vi "xc_probe.vi"() -> ()   [LabVIEW 2014]
uses:
  PIXIS_TEST/SITK_Labview/Examples70_2_2_0_1/RS Pixis/MaxY.vi
  PIXIS_TEST/SITK_Labview/Examples70_2_2_0_1/RS Pixis/MaxX.vi
  <vilib>/Analysis/Matrix/Numeric/Conversions/Array To Matrix - RA.vi
  <vilib>/Analysis/Matrix/Numeric/Conversions/Array To Matrix - RA2.vi
  <vilib>/Math Plots/3D Math Plots/3D Surface/3D Surface Datatype/Public/Plot Helper (Matrix).vi
  <vilib>/Utility/file.llb/Write To Spreadsheet File (DBL).vi
  <vilib>/Utility/file.llb/Read From Spreadsheet File (DBL).vi
  <vilib>/Analysis/Matrix/NI_Matrix.lvlib
  <vilib>/Math Plots/3D Math Plots/3D Surface/3D Surface Datatype/3D Surface Datatype.lvclass
panel:
  out "Intensity Graph":dbl[][](graph)
  in  "Background":bool=TRUE
  in  "Filter":bool=TRUE
  in  "initial parameters":dbl[](array[numeric])
  in  "?":enum16{"Lorantzian", "fano", "gaussian"}(ring)=enum."gaussian"
  in  "parameter bounds":T1={"amp min"=-inf, "amp max"=inf, "deviation min"=-inf, "deviation max"=inf, "offset min"=0.0, "offset max"=0.0}
  in  "file path":path
  in  "fit":bool
  in  "pick":bool
  in  "quit Button 2":bool
  in  "# Images":u16=200 min=2 max=10000 step=2
  in  "Flip Spectra":bool
  out "Temperature":dbl=-75.5
  out "error out":errorcluster
  out "Camera Handle":u32=16842752
  in  "error in":errorcluster
  out "Waveform Graph":dbl[](graph)
  out "Identification":string="(c)2010 Physik Instrumente(PI) Karlsruhe, C-867.160,0,1.2.0.1"
  out "PI Stage Error 2":errorcluster
  in  "PI Stage Error":errorcluster
  in  "Shutter Position":bool=TRUE
  out "Status":string="Shutter Closed"
  in  "error in2":errorcluster
  out "error out 2":errorcluster={"status"=TRUE, "code"=1097, "source"="Call Library Function Node in Shutter_Close.vi->xc_umn1.vi"}
  out "Current position":dbl=9.0349
  in  "move":bool
  in  "Start Position":dbl=9.0
  in  "Averages":u16=2
  in  "save":bool
  in  "quit Button":bool
  in  "Start Button":bool
  in  "Increment (in mm)":dbl=0.01
  in  "Range (in mm)":dbl=6.0
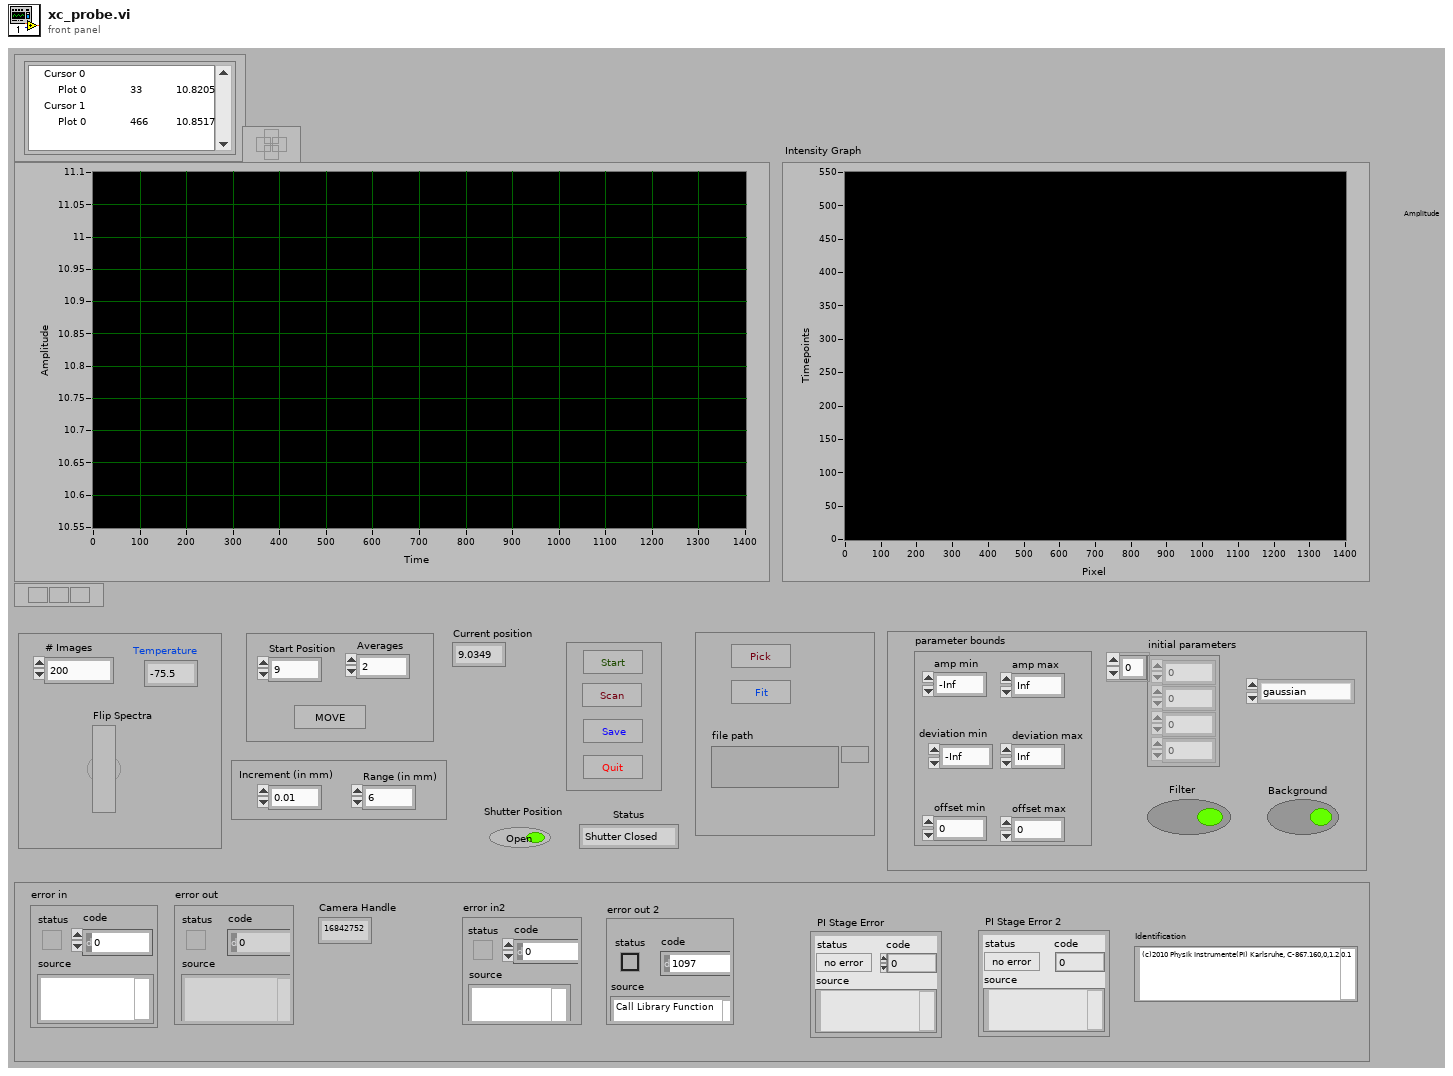
[diagram p1: front panel]
types:
  T1 = cluster{"amp min":dbl, "amp max":dbl, "deviation min":dbl, "deviation max":dbl, "offset min":dbl, "offset max":dbl}
  T2 = cluster{"X start":u32, "X end":u32, "X Binning/Grouping":u32, "Y start":u32, "Y end":u32, "Y Binning/Grouping":u32}
  T3 = typedef "NI_Matrix.lvlib/RealMatrix.ctl" = dbl[][]
  T4 = cluster{"amp min":dbl, "amp max":dbl, dbl, dbl, "deviation min":dbl, "deviation max":dbl, "offset min":dbl, "offset max":dbl}
  T5 = cluster{dbl, "result":dbl, dbl, "delta amplitude":dbl, dbl, "delta standard deviation":dbl, "center":dbl, "delta center":dbl}
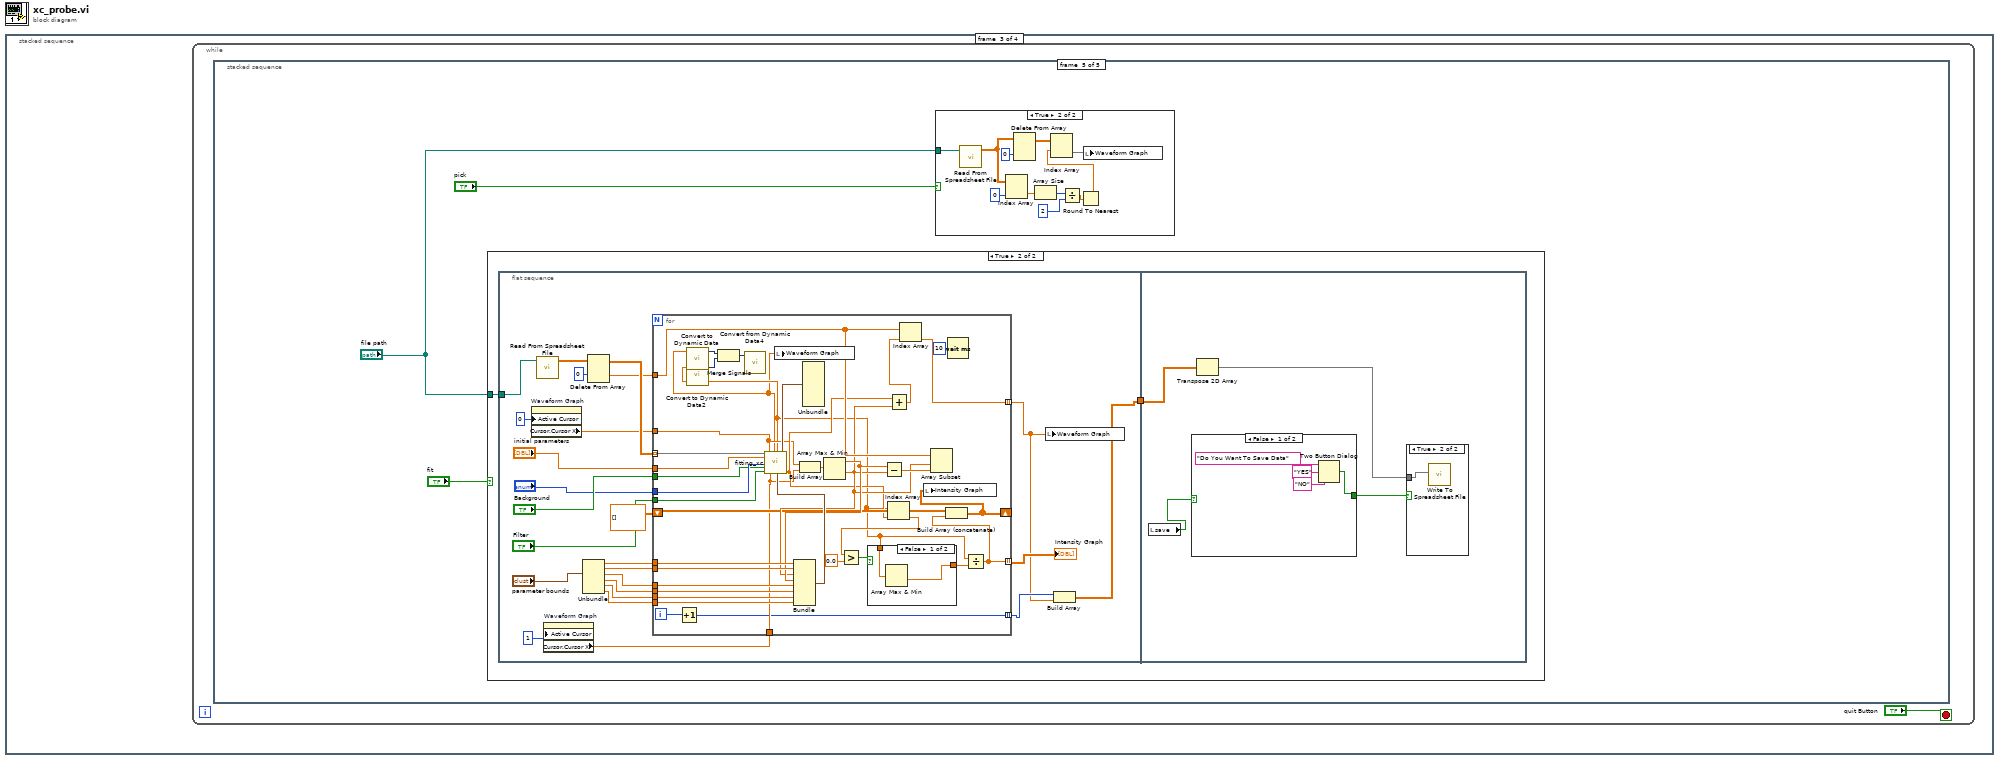
[diagram p0: block diagram]
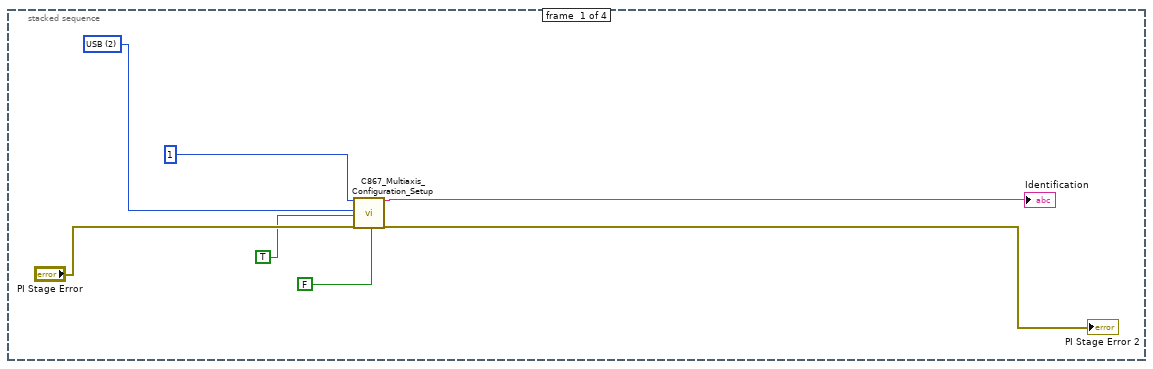
[diagram p2: hidden frame]
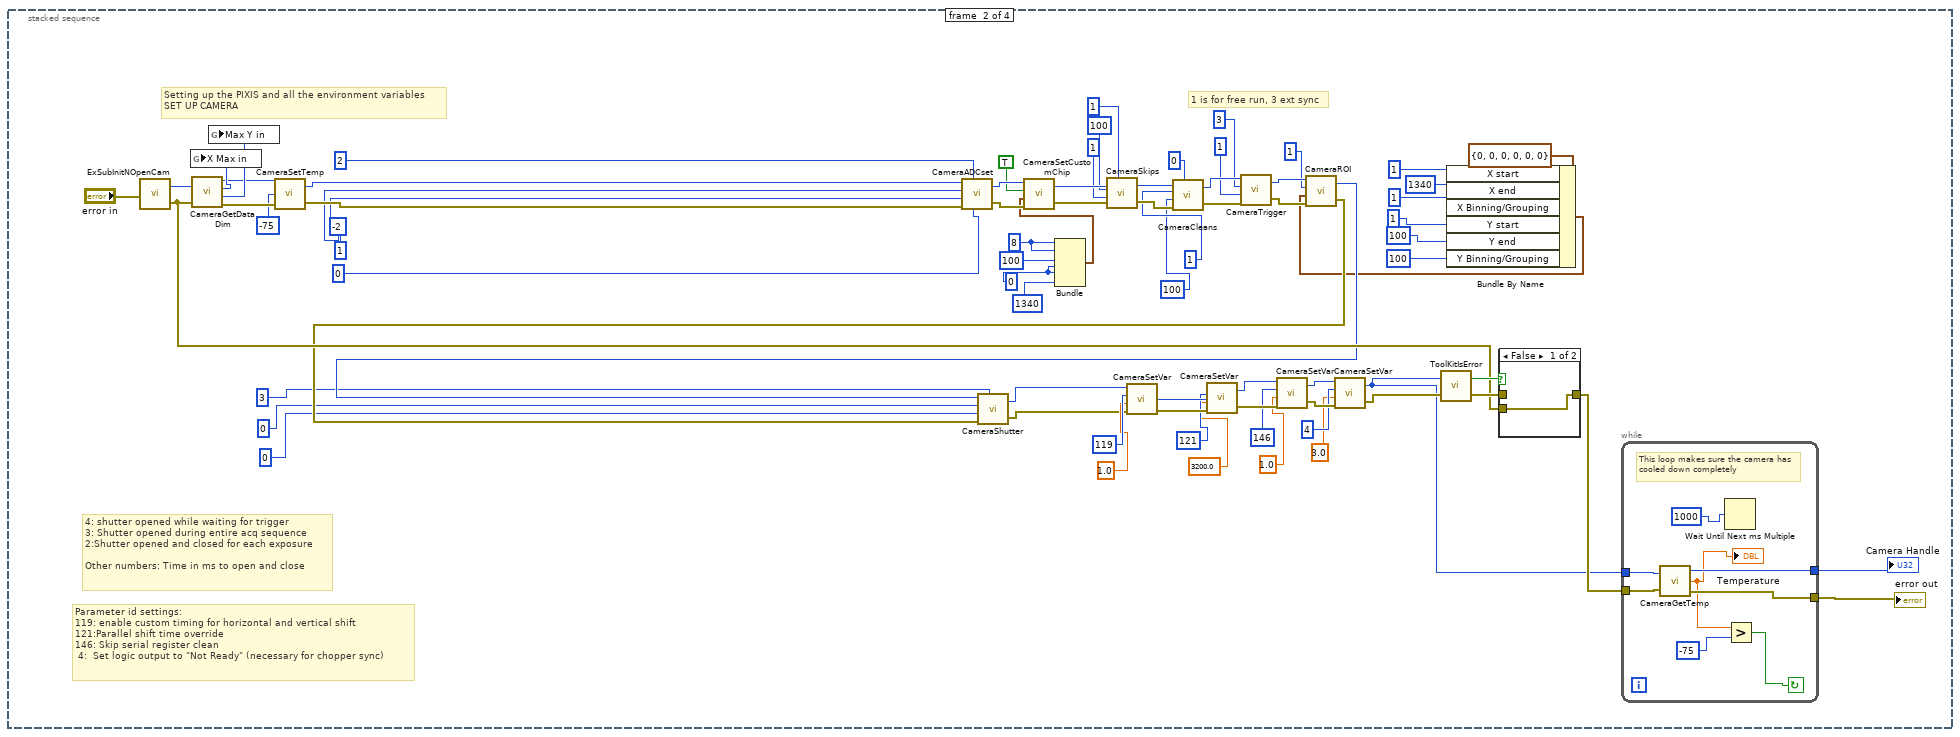
[diagram p3: hidden frame]
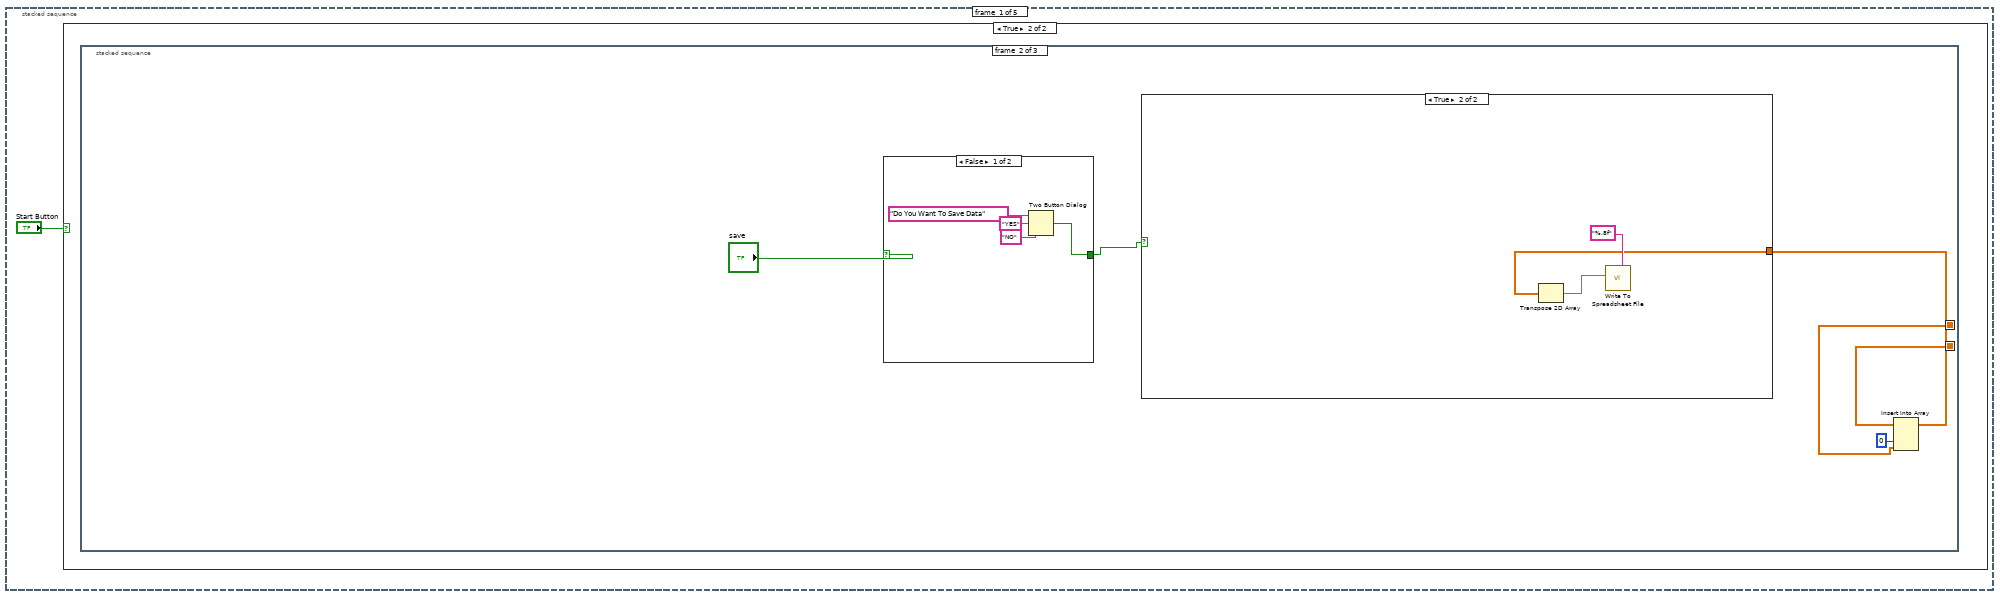
[diagram p5: hidden frame]
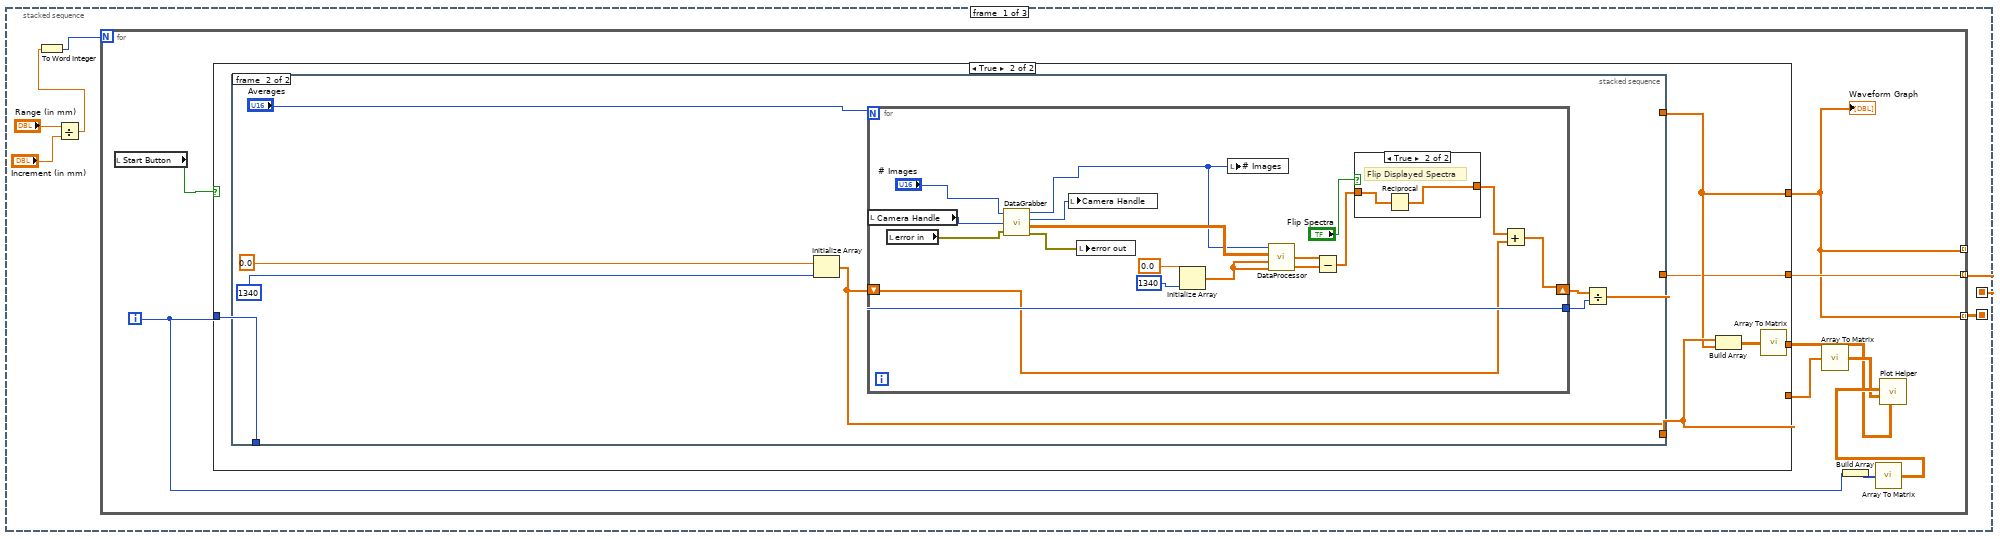
[diagram p7: hidden frame]
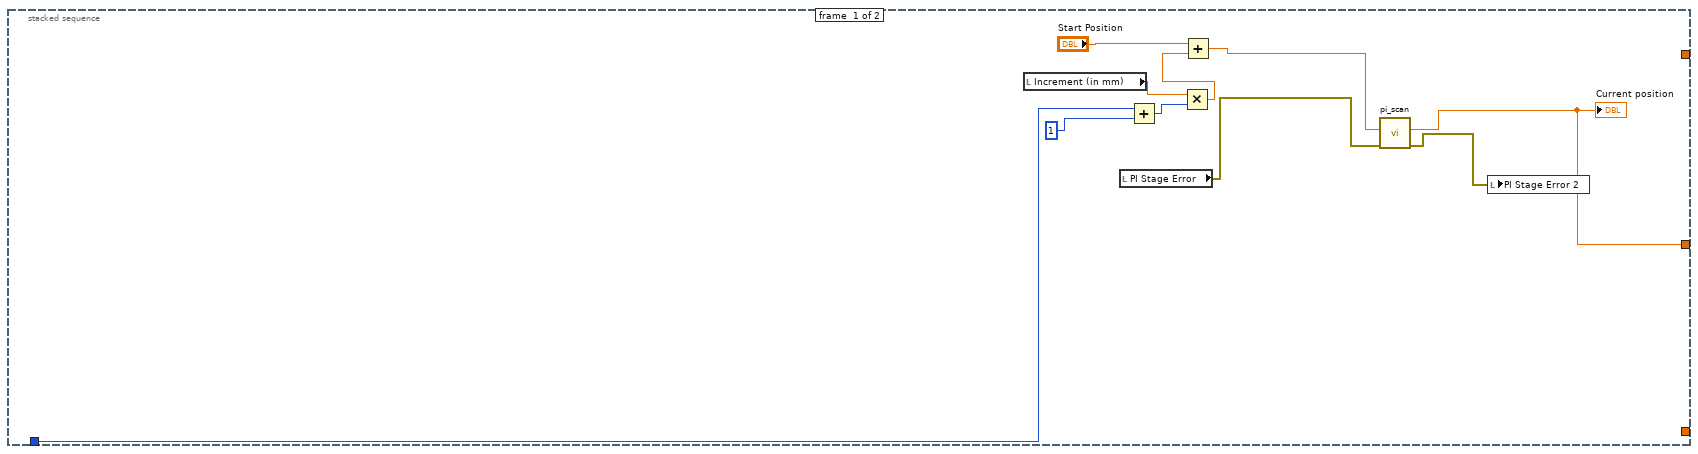
[diagram p9: hidden frame]
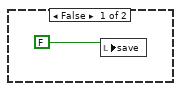
[diagram p12: hidden frame]
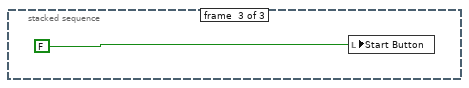
[diagram p13: hidden frame]
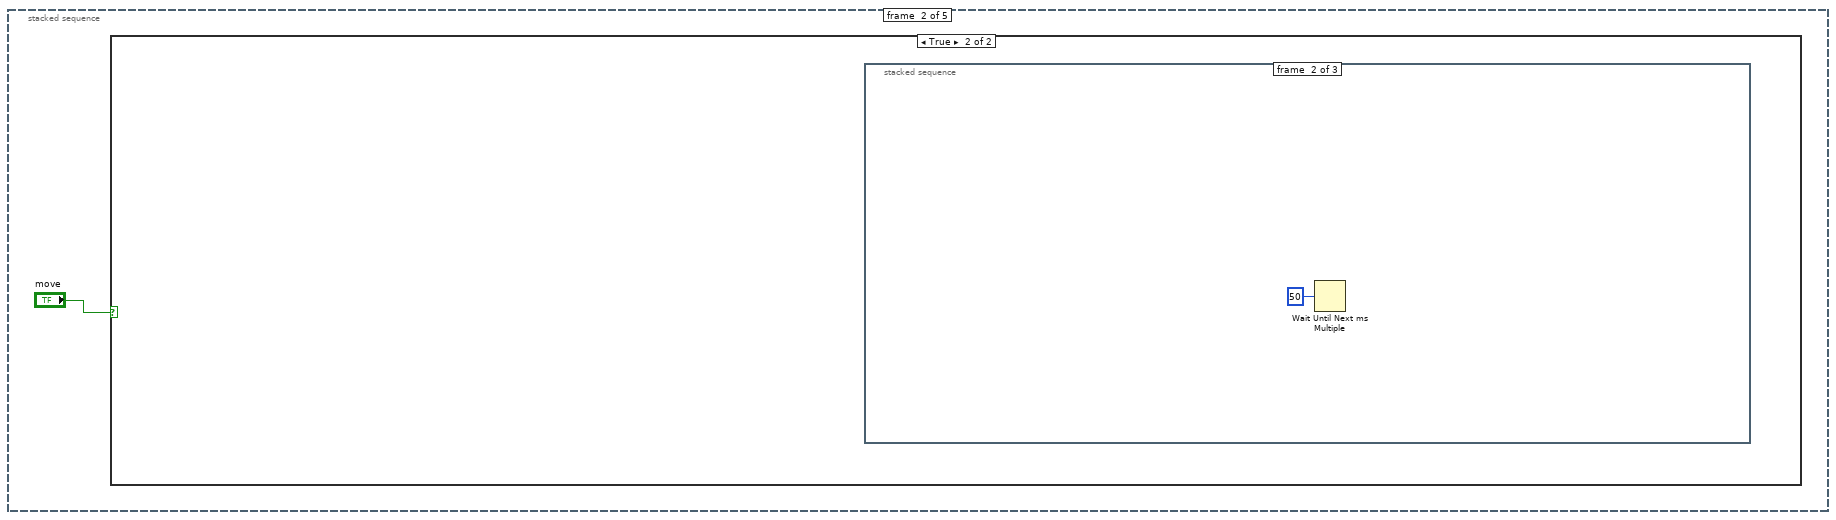
[diagram p14: hidden frame]
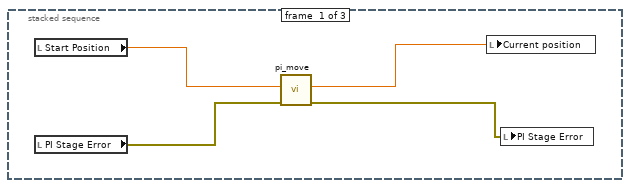
[diagram p16: hidden frame]
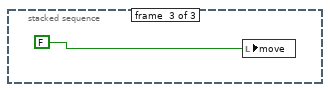
[diagram p17: hidden frame]
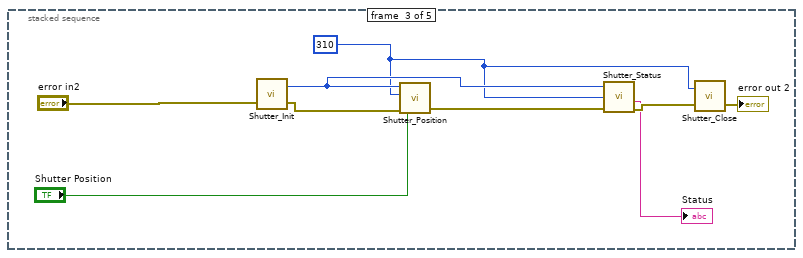
[diagram p18: hidden frame]
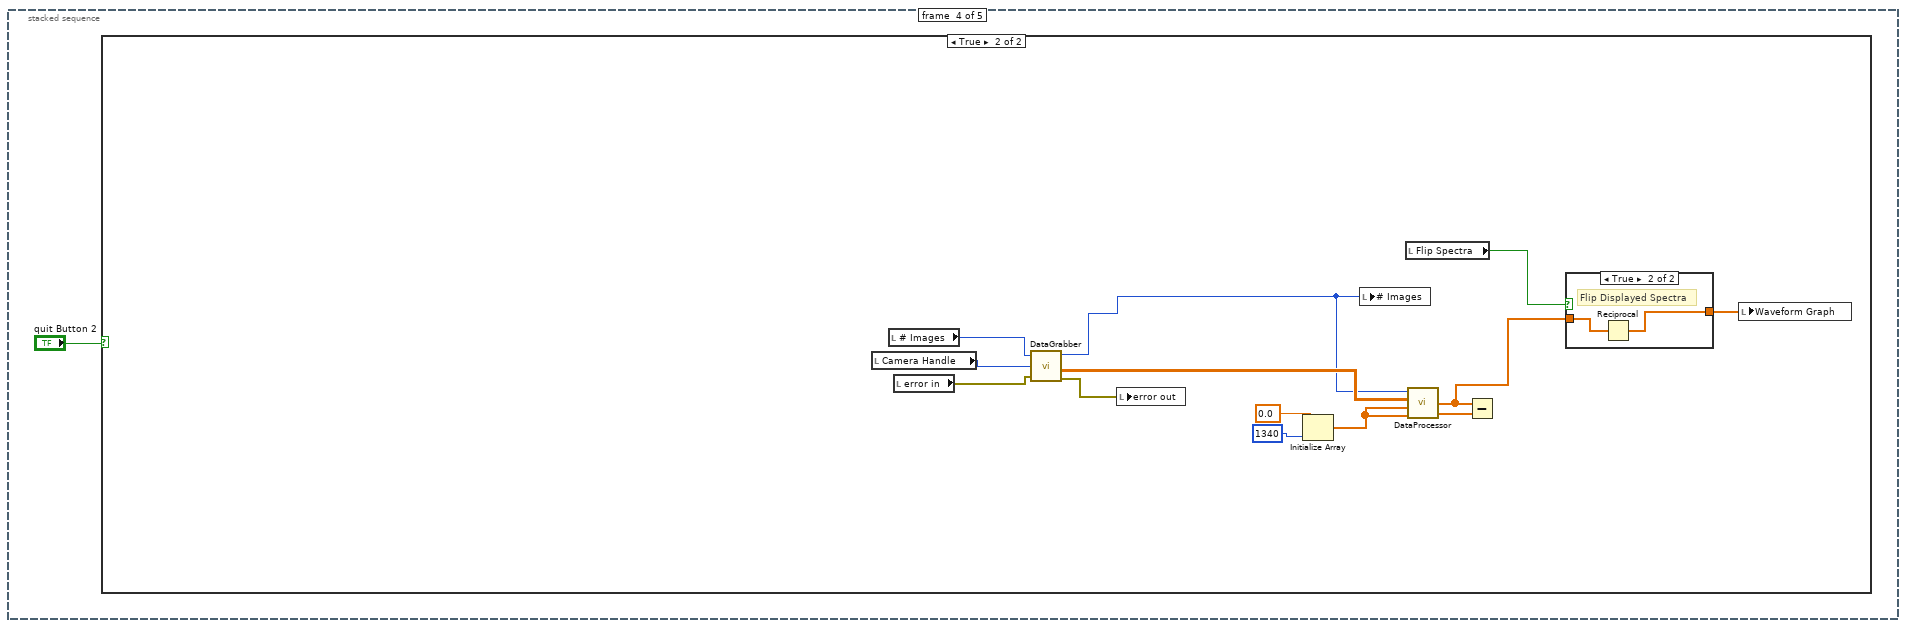
[diagram p19: hidden frame]
diagram:
  n1 = stacked-sequence {
    frame #0 {
      w4 = u16 2 items=["RS232", "RS232 DaisyChain", "USB"] ("Interface")
      n2 = call "C867_Multiaxis_Configuration_Setup.vi"("System no."=1, "Interface"=w4, "All axes?"=TRUE, "error in"="PI Stage Error", "Switch servo on?"=FALSE) -> ("Identification"=→"Identification":string, "error out"=→"PI Stage Error 2":errorcluster)  [unwired: 8 in, 5 out]
    }
    frame #1 {
      w66 = 0
      w68 = 8
      # "4: shutter opened while waiting for trigger\n3: Shutter opened during entire acq sequence\n2:Shutter opened and closed for each exposure\n\nOther numbers: Time in ms to open and close"
      # "1 is for free run, 3 ext sync"
      # "Parameter id settings:\n119: enable custom timing for horizontal and vertical shift\n121:Parallel shift time override\n146: Skip serial register clean\n 4:  Set logic output to \"Not Ready\" (necessary for chopper sync)"
      # "Setting up the PIXIS and all the environment variables\nSET UP CAMERA"
      n3 = call "ExSubInitNOpenCam.vi"("error in (no error)"="error in") -> ("Camera Handle"=w81:u32, "error out"=w38:errorcluster)
      n4 = call <userlib>:"CameraGetDataDim.vi"("Camera Handle"=w81, "error in"=w38) -> ("Camera Handle"=w78:u32, "Xdim"=w80:u32, "Ydim"=w79:u32, "error out"=w77:errorcluster)
      n5 = global write "MaxX.vi" "X Max in"(w80) -> ()
      n6 = global write "MaxY.vi" "Max Y in"(w79) -> ()
      n7 = call <userlib>:"CameraSetTemp.vi"("error in (no error)"=w77, "Temperature"=-75, "Camera Handle"=w78) -> ("error out"=w74:errorcluster, "Camera Handle"=w75:u32)
      n8 = call <userlib>:"CameraADCset.vi"("ADC offset"=0, "Read Out port"=2, "error in (no error)"=w74, "ADC Gain"=1, "ADC Speed"=-2, "Camera Handle"=w75) -> ("error out"=w69:errorcluster, "Camera Handle"=w70:u32)
      n9 = Bundle(w68, w68, 100, w66, w66, 1340) -> (w65:cluster{i32, i32, i32, i32, i32, i32})  [unwired: 1 in]
      n10 = call <userlib>:"CameraSetCustomChip.vi"("error in (no error)"=w69, "Custom Chip Settings"=w65, "Enable/Disable Custom Chip"=TRUE, "Camera Handle"=w70) -> ("error out"=w62:errorcluster, "Camera Handle"=w63:u32)
      n11 = call <userlib>:"CameraSkips.vi"("Camera Handle"=w63, "Minimum Block Size"=100, "Number of Minimum blocks"=1, "error in"=w62, "Type of Skips"=1) -> ("Camera Handle"=w57:u32, "error out"=w58:errorcluster)
      n12 = call <userlib>:"CameraCleans.vi"("Camera Handle"=w57, "Number of Clears"=1, "Number of Strips Per Clear"=100, "error in"=w58, "Continuous Clears"=0) -> ("Camera Handle"=w52:u32, "error out"=w53:errorcluster)
      n13 = call <userlib>:"CameraTrigger.vi"("error in"=w53, "Trigger Edge"=1, "Timing Mode"=3, "Camera Handle"=w52) -> ("error out"=w30:errorcluster, "Camera Handle"=w29:u32)
      n14 = Bundle By Name(cluster=T2 {"X start"=0, "X end"=0, "X Binning/Grouping"=0, "Y start"=0, "Y end"=0, "Y Binning/Grouping"=0} ("ROI Params"), "X start"=u32 1, "X end"=u32 1340, "X Binning/Grouping"=u32 1, "Y start"=u32 1, "Y end"=u32 100, "Y Binning/Grouping"=u32 100) -> (w11:T2)
      n15 = call <userlib>:"CameraROI.vi"("error in"=w30, "ROI Params"=w11, "ROI Index"=1, "Camera Handle"=w29) -> ("error out"=w24:errorcluster, "Camera Handle"=w23:u32)
      n16 = call <userlib>:"CameraShutter.vi"("Camera Handle"=w23, "Shutter Comp Time: Pre Open"=0, "Shutter Comp Time: Post Open"=0, "error in"=w24, "Shutter State"=3) -> ("Camera Handle"=w22:u32, "error out"=w13:errorcluster)
      n17 = call <userlib>:"CameraSetVar.vi"("error in"=w13, "Value"=1.0, "Parameter ID"=119, "Camera Handle"=w22) -> ("error out"=w47:errorcluster, "CameraHandle"=w45:u32)
      n18 = call <userlib>:"CameraSetVar.vi"("error in"=w47, "Value"=3200.0, "Parameter ID"=121, "Camera Handle"=w45) -> ("error out"=w46:errorcluster, "CameraHandle"=w44:u32)
      n19 = call <userlib>:"CameraSetVar.vi"("error in"=w46, "Value"=1.0, "Parameter ID"=146, "Camera Handle"=w44) -> ("error out"=w18:errorcluster, "CameraHandle"=w17:u32)
      n20 = call <userlib>:"CameraSetVar.vi"("error in"=w18, "Value"=3.0, "Parameter ID"=4, "Camera Handle"=w17) -> ("error out"=w16:errorcluster, "CameraHandle"=w9:u32)
      n21 = call <userlib>:"ToolKitIsError.vi"("error in"=w16, "Reserved"=w9) -> ("error out"=w48:errorcluster, "Error Flag"=w49:bool)
      n22 = case shown="False" w49 {
        tunnel: w48 -> [_ w92]
        tunnel: [w91 w92] -> w10
        tunnel: w38 -> [w91 _]
        frame False {
        }
        frame True {
        }
      }
      n23 = while {
        tunnel: w10 -> [w89]
        tunnel: [w88] -> w26
        tunnel: w9 -> [w87]
        tunnel: [w86] -> w27
        stop <- w84 continue-if-true
        # "This loop makes sure the camera has cooled down completely"
        n24 = call <userlib>:"CameraGetTemp.vi"("Camera Handle"=w87, "error in (no error)"=w89) -> ("Camera Handle"=w86:u32, "Temperature"=w83:dbl, "error out"=w88:errorcluster)
        "Temperature" <- w83
        n25 = Wait Until Next ms Multiple(millisecond multiple=1000 ("ADC Gain")) -> ()  [unwired: 1 out]
        n26 = Greater?(x=w83, y=-75) -> (0:w84:bool)
      }
      "Camera Handle" <- w27
      "error out" <- w26
    }
    frame #2 {
      n27 = while {
        stop <- "quit Button" stop-if-true
        n28 = stacked-sequence {
          frame #0 {
            n29 = case shown="True" "Start Button" {
              frame False {
              }
              frame True {
                n30 = stacked-sequence {
                  seq-local: [w96 _ _] -> [_ w155 _]
                  seq-local: [w95 _ _] -> [_ w157 _]
                  frame #0 {
                    n31 = Divide(x="Range (in mm)", y="Increment (in mm)") -> (x/y=w98:dbl)
                    n32 = To Word Integer(number=w98) -> (16bit integer=w97:i16)
                    n33 = for {
                      N: w97 -> [_]
                      tunnel: [w101] -> _ mode=indexing
                      tunnel: [w102] -> w96 mode=indexing
                      tunnel: [w101] -> w95 mode=indexing
                      i -> [w108]
                      n34 = local read "Start Button"() -> (w109:bool)
                      n35 = case shown="True" w109 {
                        tunnel: w108 -> [_ w115]
                        tunnel: [_ w114] -> w105
                        tunnel: [_ w112] -> w103
                        tunnel: [_ w111] -> w101
                        tunnel: [_ w110] -> w102
                        frame False {
                        }
                        frame True {
                          n36 = stacked-sequence {
                            tunnel: w115 -> [w120 _]
                            tunnel: [_ w126] -> w111
                            tunnel: [_ w127] -> w114
                            tunnel: [w116 _] -> w110
                            frame #0 {
                              n37 = local read "Increment (in mm)"() -> (w122:dbl)
                              n38 = local read "PI Stage Error"() -> (w118:errorcluster)
                              n39 = Add(x=w120, y=1) -> (x+y=w123:i32)
                              n40 = Multiply(x=w122, y=w123) -> (x*y=w124:dbl)
                              n41 = Add(x="Start Position", y=w124) -> (x+y=w119:dbl)
                              n42 = call "pi_scan.vi"("error in"=w118, "Start Position"=w119) -> ("error out"=w117:errorcluster, "element"=w116:dbl)  [unwired: 8 in]
                              "Current position" <- w116
                              n43 = local write "PI Stage Error 2"(w117) -> ()
                            }
                            frame #1 {
                              n44 = Initialize Array(0.0 ("element"), 1340 ("dimension size")) -> (w127:dbl[])
                              n45 = for {
                                N: "Averages" -> [w140]
                                shift-right: [w138] -> w131
                                shift-left: w127 -> [w137]
                                tunnel: [w140] -> w130
                                n46 = local read "Camera Handle"() -> (w150:u32)
                                n47 = local read "error in"() -> (w149:errorcluster)
                                n48 = call "DataGrabber.vi"("# Images In"="# Images", "Camera Handle"=w150, "error in (no error)"=w149) -> ("# Images Out"=w143:u16, "Camera Handle"=w148:u32, "Data"=w144:dbl[][], "error out"=w141:errorcluster)
                                n49 = local write "Camera Handle"(w148) -> ()
                                n50 = local write "error out"(w141) -> ()
                                n51 = Initialize Array(0.0, u32 1340) -> (w146:dbl[])
                                n52 = local write "# Images"(w143) -> ()
                                n53 = call "DataProcessor.vi"("PumpOffBkgd"=w146, "PumpOnBkgd"=w146, "Data"=w144, "# of Images"=w143) -> ("PumpOff"=w134:dbl[], "PumpOn"=w135:dbl[])  [unwired: 1 out]
                                n54 = Subtract(x=w135, y=w134) -> (x-y=w133:dbl[])
                                n55 = case shown="True" "Flip Spectra" {
                                tunnel: [w151 w152] -> w139
                                tunnel: w133 -> [w151 w153]
                                frame False {
                                }
                                frame True {
                                # "Flip Displayed Spectra"
                                n56 = Reciprocal(x=w153) -> (1/x=w152:dbl[])
                                }
                                }
                                n57 = Add(x=w139, y=w137) -> (x+y=w138:dbl[])
                              }
                              n58 = Divide(x=w131, y=w130) -> (x/y=w126:dbl[])
                            }
                          }
                          n59 = Build Array(w114, w111) -> (w113:dbl[][])
                          n60 = call-poly <vilib>:"Array To Matrix.vi"("Real 2D Array"=w113) -> ("Real Matrix"=w112:T3)
                        }
                      }
                      "Waveform Graph" <- w101
                      n61 = call-poly <vilib>:"Array To Matrix.vi"("Real 1D Array"=w105) -> ("Real Matrix (Column Vector)"=w104:T3)
                      n62 = Build Array(w108) -> (w107:i32[])
                      n63 = call-poly <vilib>:"Array To Matrix.vi"("Real 1D Array"=w107) -> ("Real Matrix (Column Vector)"=w106:T3)
                      n64 = call-poly <vilib>:"Plot Helper.vi"("z matrix"=w103, "y matrix"=w104, "x matrix"=w106) -> ()  [unwired: 3 in, 6 out]
                    }
                  }
                  frame #1 {
                    n65 = case shown="False" "save" {
                      selector: "save" -> [_ w164]
                      tunnel: [w160 w164] -> w158
                      frame False {
                        n66 = Two Button Dialog(message="Do You Want To Save Data", 1:"NO" ("F button name (\"Cancel\")"), 2:"YES" ("T button name (\"OK\")")) -> (T button?=w160:bool)
                      }
                      frame True {
                      }
                    }
                    n67 = Insert Into Array(array=w157, index (col)=0 ("disabled index (col)"), new element=w155) -> (w154:dbl[][])  [unwired: 1 in]
                    n68 = case shown="True" w158 {
                      tunnel: w154 -> [_ w167]
                      frame False {
                        n69 = local write "save"(FALSE) -> ()
                      }
                      frame True {
                        n70 = Transpose 2D Array(2D array=w167) -> (transposed array=w166:dbl[][])
                        n71 = call-poly <vilib>:"Write To Spreadsheet File.vi"("format (%.3f)"="%.8f", "2D data"=w166) -> ()  [unwired: 6 in, 1 out]
                      }
                    }
                  }
                  frame #2 {
                    n72 = local write "Start Button"(FALSE) -> ()
                  }
                }
              }
            }
          }
          frame #1 {
            n73 = case shown="True" "move" {
              frame False {
              }
              frame True {
                n74 = stacked-sequence {
                  frame #0 {
                    n75 = local read "Start Position"() -> (w174:dbl)
                    n76 = local read "PI Stage Error"() -> (w173:errorcluster)
                    n77 = call "pi_move.vi"("error in"=w173, "Start Position"=w174) -> ("error out"=w172:errorcluster, "element"=w171:dbl)  [unwired: 8 in]
                    n78 = local write "Current position"(w171) -> ()
                    n79 = local write "PI Stage Error"(w172) -> ()
                  }
                  frame #1 {
                    n80 = Wait Until Next ms Multiple(millisecond multiple=u32 50) -> ()  [unwired: 1 out]
                  }
                  frame #2 {
                    n81 = local write "move"(FALSE) -> ()
                  }
                }
              }
            }
          }
          frame #2 {
            w178 = 310
            n82 = call "Shutter_Init.vi"("error in"="error in2") -> ("error out"=w183:errorcluster, "ObjectPtr"=w180:i32)  [unwired: 1 in]
            n83 = call "Shutter_Position.vi"("error in"=w183, "Shutter Position"="Shutter Position", "ShutterID"=w178, "ObjectPtr"=w180) -> ("error out"=w182:errorcluster)  [unwired: 2 in]
            n84 = call "Shutter_Status.vi"("ObjectPtr"=w180, "ShutterID"=w178, "error in"=w182) -> ("Status"=→"Status":string, "error out"=w181:errorcluster)  [unwired: 2 out]
            n85 = call "Shutter_Close.vi"("error in"=w181, "ObjectPtr"=w178) -> ("error out"=→"error out 2":errorcluster)  [unwired: 1 in]
          }
          frame #3 {
            n86 = case shown="True" "quit Button 2" {
              frame False {
              }
              frame True {
                n87 = local read "Camera Handle"() -> (w198:u32)
                n88 = local read "# Images"() -> (w199:u16)
                n89 = local read "error in"() -> (w197:errorcluster)
                n90 = call "DataGrabber.vi"("# Images In"=w199, "Camera Handle"=w198, "error in (no error)"=w197) -> ("# Images Out"=w192:u16, "Data"=w193:dbl[][], "error out"=w191:errorcluster)  [unwired: 1 out]
                n91 = local write "error out"(w191) -> ()
                n92 = Initialize Array(0.0, u32 1340) -> (w195:dbl[])
                n93 = local write "# Images"(w192) -> ()
                n94 = local read "Flip Spectra"() -> (w190:bool)
                n95 = call "DataProcessor.vi"("PumpOffBkgd"=w195, "PumpOnBkgd"=w195, "Data"=w193, "# of Images"=w192) -> ("PumpOff"=w188:dbl[], "PumpOn"=w187:dbl[])  [unwired: 1 out]
                n96 = Subtract(x=w187, y=w188) -> ()  [unwired: 1 out]
                n97 = case shown="True" w190 {
                  tunnel: [w200 w201] -> w189
                  tunnel: w187 -> [w200 w202]
                  frame False {
                  }
                  frame True {
                    # "Flip Displayed Spectra"
                    n98 = Reciprocal(x=w202) -> (1/x=w201:dbl[])
                  }
                }
                n99 = local write "Waveform Graph"(w189) -> ()
              }
            }
          }
          frame #4 {
            n100 = case shown="True" "fit" {
              tunnel: "file path" -> [_ w207]
              frame False {
              }
              frame True {
                n101 = flat-sequence {
                  tunnel: w207 -> [w216]
                  tunnel: [w208] -> w206
                  tunnel: w206 -> [w276]
                  frame #0 {
                    n102 = property on="Waveform Graph" class="WFGraph (strict)"("Active Cursor"=u32 0) -> ("Cursor.Cursor X"=w211:dbl)  [unwired: 2 in, 2 out]
                    n103 = call-poly <vilib>:"Read From Spreadsheet File.vi"("file path (dialog if empty)"=w216) -> ("all rows"=w232:dbl[][])  [unwired: 6 in, 4 out]
                    n104 = property on="Waveform Graph" class="WFGraph (strict)"("Active Cursor"=u32 1) -> ("Cursor.Cursor X"=w213:dbl)  [unwired: 2 in, 2 out]
                    n105 = Unbundle("parameter bounds") -> ("amp min"=w229:dbl, "amp max"=w228:dbl, "deviation min"=w227:dbl, "deviation max"=w226:dbl, "offset min"=w225:dbl, "offset max"=w224:dbl)
                    n106 = Delete From Array(array=w232, index (row)=0) -> (deleted portion=w223:dbl[], array with subset deleted=w230:dbl[][])  [unwired: 2 in]
                    n107 = for {
                      tunnel: w230 -> [w256] mode=indexing
                      tunnel: "initial parameters" -> [w270]
                      tunnel: "?" -> [w269]
                      tunnel: "Background" -> [w268]
                      tunnel: "Filter" -> [w267]
                      tunnel: w229 -> [w266]
                      tunnel: w228 -> [w265]
                      tunnel: w227 -> [w264]
                      tunnel: w226 -> [w263]
                      tunnel: w225 -> [w262]
                      tunnel: w224 -> [w261]
                      tunnel: [w235] -> w209 mode=indexing
                      tunnel: w223 -> [w252]
                      tunnel: [w243] -> w215 mode=indexing
                      shift-right: [w240] -> _
                      shift-left: dbl[][] [] -> [w245]
                      tunnel: w213 -> [w239]
                      tunnel: w211 -> [w238]
                      tunnel: [w233] -> w210 mode=indexing
                      i -> [w234]
                      n108 = Increment(x=w234) -> (x+1=w233:i32)
                      n109 = Build Array(w238, w239) -> (w260:dbl[])
                      n110 = Array Max & Min(array=w260) -> (max value=w251:dbl, min value=w250:dbl)  [unwired: 2 out]
                      n111 = Bundle("amp min"=w266, "amp max"=w265, w250, w251, "deviation min"=w264, "deviation max"=w263, "offset min"=w262, "offset max"=w261) -> (w259:T4)  [unwired: 1 in]
                      n112 = call "fitting_xc.vi"("array"=w256, "initial parameters"=w270, "Enum"=w269, "Background"=w268, "Filter"=w267, "x"=w238, "x 2"=w239, "parameter bounds"=w259) -> ("sub_Y"=w236:dbl[], "Best Gaussian Fit"=w237:dbl[], "output cluster"=w258:T5, "center"=w244:dbl)  [unwired: 6 in, 2 out]
                      n113 = call "Convert to Dynamic Data"("Array"=w236) -> ("Dynamic Data Type"=w255:dynamicdata)  [unwired: 3 in]
                      n114 = call "Convert to Dynamic Data2"("Array"=w237) -> ("Dynamic Data Type"=w254:dynamicdata)  [unwired: 3 in]
                      n115 = Merge Signals(w255, w254) -> (w241:dynamicdata)
                      n116 = call "Convert from Dynamic Data4"("Dynamic Data Type"=w241) -> ()  [unwired: 3 in, 1 out]
                      n117 = local write "Waveform Graph"(w236) -> ()
                      n118 = Unbundle(w258) -> ()  [unwired: 8 out]
                      n119 = Subtract(x=w251, y=w250) -> (x-y=w253:dbl)
                      n120 = Index Array(array=w237, index=w244) -> (element=w248:dbl)
                      n121 = Greater?(x=w248, y=0.0) -> (0:w247:bool)
                      n122 = case shown="False" w247 {
                        tunnel: w237 -> [w271 w274]
                        tunnel: [w272 w273] -> w246
                        frame False {
                          n123 = Array Max & Min(array=w271) -> (min value=w272:dbl)  [unwired: 3 out]
                        }
                        frame True {
                          n124 = Array Max & Min(array=w274) -> (max value=w273:dbl)  [unwired: 3 out]
                        }
                      }
                      n125 = Add(x=w244, y=w250) -> (x+y=w257:dbl)
                      n126 = Index Array(array=w252, index=w257) -> (element=w235:dbl)
                      n127 = Array Subset(array=w252, index=w250, length=w253) -> ()  [unwired: 1 out]
                      n128 = Wait (ms)(milliseconds to wait=u32 10) -> ()  [unwired: 1 out]
                      n129 = Divide(x=w237, y=w246) -> (x/y=w243:dbl[])
                      n130 = Build Array (concatenate)(w245, w243) -> (w240:dbl[][])
                      n131 = local write "Intensity Graph"(w240) -> ()
                    }
                    "Intensity Graph" <- w215
                    n132 = local write "Waveform Graph"(w209) -> ()
                    n133 = Build Array(w210, w209) -> (w208:dbl[][])
                  }
                  frame #1 {
                    n134 = local read "save"() -> (w277:bool)
                    n135 = case shown="False" w277 {
                      selector: w277 -> [_ w284]
                      tunnel: [w280 w284] -> w278
                      frame False {
                        n136 = Two Button Dialog(message="Do You Want To Save Data", 1:"NO" ("F button name (\"Cancel\")"), 2:"YES" ("T button name (\"OK\")")) -> (T button?=w280:bool)
                      }
                      frame True {
                      }
                    }
                    n137 = Transpose 2D Array(2D array=w276) -> (transposed array=w275:dbl[][])
                    n138 = case shown="True" w278 {
                      tunnel: w275 -> [_ w279]
                      frame False {
                      }
                      frame True {
                        n139 = call-poly <vilib>:"Write To Spreadsheet File.vi"("2D data"=w279) -> ()  [unwired: 7 in, 1 out]
                      }
                    }
                  }
                }
              }
            }
            n140 = case shown="True" "pick" {
              tunnel: "file path" -> [_ w295]
              frame False {
              }
              frame True {
                n141 = call-poly <vilib>:"Read From Spreadsheet File.vi"("file path (dialog if empty)"=w295) -> ("all rows"=w289:dbl[][])  [unwired: 6 in, 4 out]
                n142 = Index Array(array=w289, index (col)=0 ("disabled index (col)")) -> (element=w293:dbl[])  [unwired: 1 in]
                n143 = Delete From Array(array=w289, index (row)=0) -> (array with subset deleted=w288:dbl[][])  [unwired: 2 in, 1 out]
                n144 = Array Size(array=w293) -> (size(s)=w292:i32)
                n145 = Divide(x=w292, y=2) -> (x/y=w286:dbl)
                n146 = Round To Nearest(number=w286) -> (nearest integer value=w285:dbl)
                n147 = Index Array(array=w288, index (row)=w285) -> (element=w287:dbl[])  [unwired: 1 in]
                n148 = local write "Waveform Graph"(w287) -> ()
              }
            }
          }
        }
      }
    }
    frame #3 {
      n149 = local read "PI Stage Error"() -> (w301:errorcluster)
      n150 = call "Close connection if open.vi"("System no."=1, "error in"=w301) -> ("error out"=w300:errorcluster)  [unwired: 16 in, 1 out]
      n151 = local read "Camera Handle"() -> (w296:u32)
      n152 = local write "PI Stage Error 2"(w300) -> ()
      n153 = local read "error in"() -> (w297:errorcluster)
      n154 = call <userlib>:"CameraClose.vi"("error in"=w297, "Camera Handle"=w296) -> ("error out"=w299:errorcluster)
      n155 = call <userlib>:"UninitToolkit.vi"("error in"=w299) -> ("error out"=w298:errorcluster)
      n156 = local write "error out"(w298) -> ()
    }
  }
